vi "FlexRIO_CPUIMAQ.vi"() -> ()   [LabVIEW 2013]
uses:
  <vilib>/rvi/Emulation/niFpgaSctlEmulationGetInTimedLoop.vi
  <vilib>/rvi/Emulation/niFpgaEmulationReportErrorSimple.vi
  <vilib>/rvi/Emulation/niFpgaGetClockAttributes.vi
  <vilib>/rvi/interface/RandomDataEmulation/nirviRandomDataFPGAFIFO.vi
  <vilib>/rvi/interface/RandomDataEmulation/niFpgaRandomDataHandleErrors.vi
  <vilib>/rvi/Emulation/niFpgaCriticalErrorInLSC.vi
  <vilib>/rvi/DataTransferAndStorage/Container/XNode/niFpgaContainer.xnode
  <vilib>/rvi/interface/RandomDataEmulation/nirviRandomDataFpgaReadWriteTemplate.vi
panel:
  out "uartOverrunError":bool
  out "uartFramingError":bool
  out "uartBreakIndicator":bool
  out "uartRxByte":u8 format="%02x"
  out "uartTxReady":bool
  out "uartRxReady":bool
  in  "uartTxByte":u8=1 format="%x"
  in  "uartByteMode":bool=TRUE
  in  "uartBaudRate":u8=1
  in  "uartSetBaudRate":bool
  in  "uartReceive":bool
  in  "uartTransmit":bool
  in  "ControlEnable":bool=TRUE
  in  "LineScan":bool
  in  "SpareHigh":bool=TRUE
  in  "LVALHigh":bool=TRUE
  in  "FVALHigh":bool=TRUE
  in  "DVALHigh":bool=TRUE
  in  "SignalMapping":u8(ring) items=["Standard", "Basler 10 tap", "Vosskühler 10 tap"]
  in  "Configuration":u8(ring)=2 items=["Base", "Medium", "Full/Extended"]
  out "PXIIN1":bool
  in  "PXIOUT1":bool
  out "PXIIN0":bool
  in  "PXIOUT0":bool
  out "auxDI1":bool
  out "auxDI0":bool
  out "DI1":bool
  out "DI0":bool
  in  "auxDO1":bool
  in  "auxDO0":bool
  in  "DO1":bool
  in  "DO0":bool
  in  "auxAO1":i32
  in  "auxAO0":i32
  out "auxAI1":i32
  out "auxAI0":i32
  out "DMATtoHOSTOverflows":u16
  in  "DMATtoHOSTEnable0":bool
  out "DMATtoHOSTSampleSize":u8[](array[numeric])
  out "DMATtoHOSTFrameType":u8[](array[numeric])
  out "DMATtoHOSTNCh":u16[](array[numeric])
  out "Platform":enum8{"FlexRIO", "cRIO", "RSeries"}(ring)
  in  "DebugMode":bool
  in  "DAQStartStop":bool
  out "DevProfile":T1(ring)=enum."CPUImage"
  out "DevTemp":i16=-10244
  out "DevQualityStatus":u8
  out "Fref":u32=100000000
  out "RIOAdapterCorrect":bool=TRUE
  out "InsertedIOModule ID":u32
  out "InitDone":bool=TRUE
  out "FPGAVIversion":u8[](array[numeric])=[1, 0]
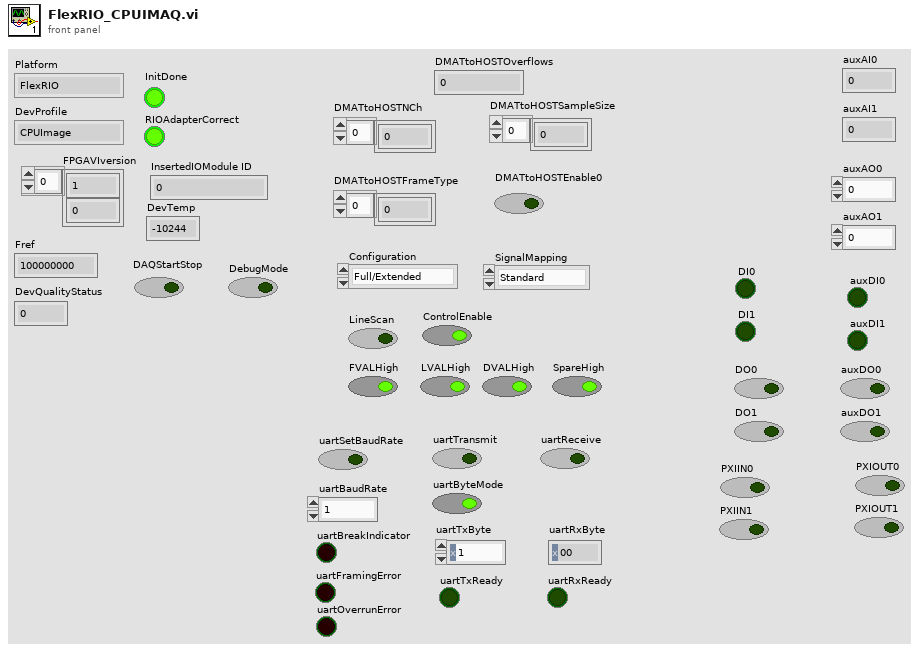
[diagram p1: front panel]
types:
  T1 = enum8{"CPUData", "CPUImage", "GPUData", "GPUImage"}
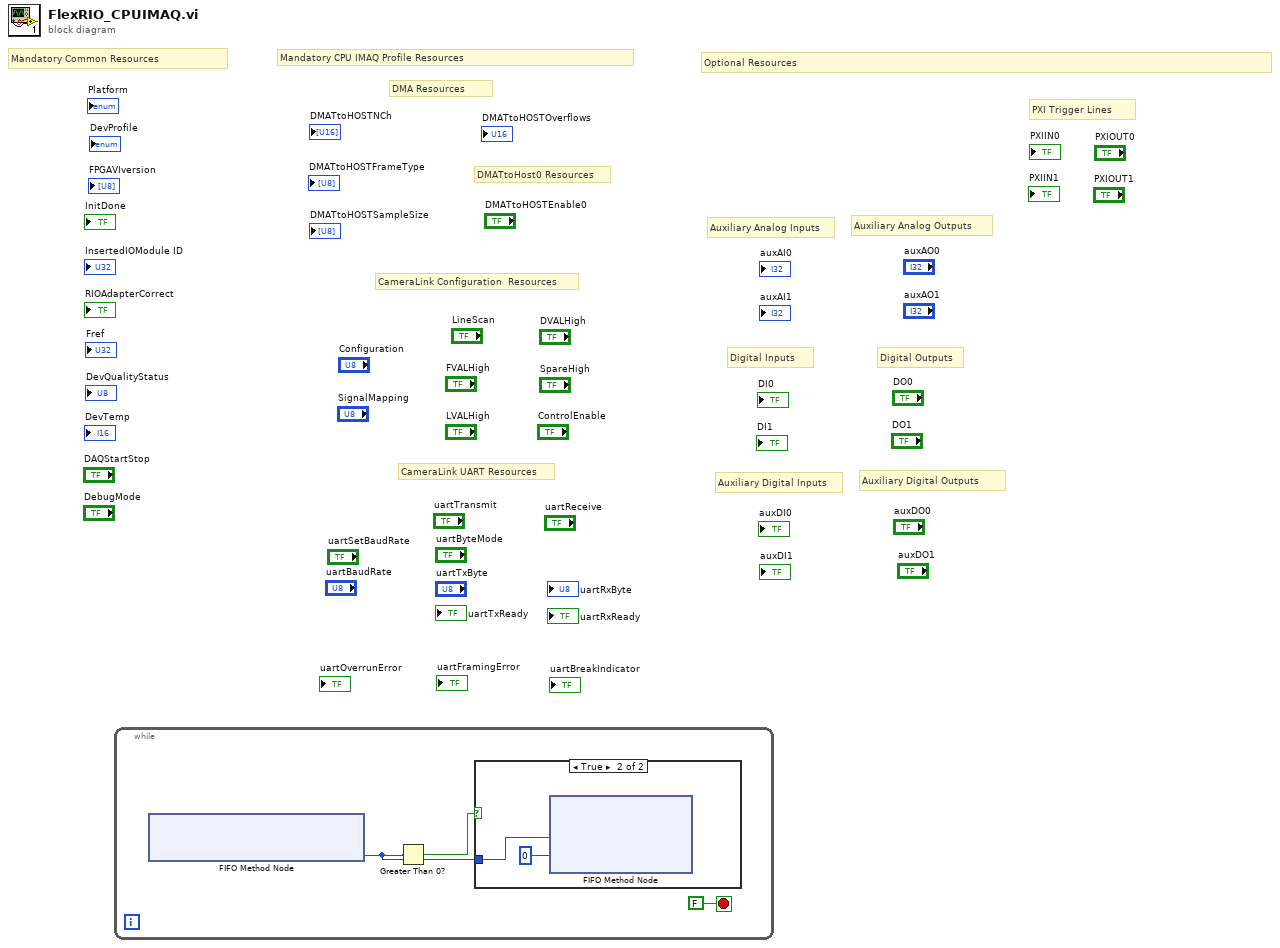
[diagram p0: block diagram]
diagram:
  # "CameraLink UART Resources"
  # "CameraLink Configuration  Resources"
  # "DMA Resources"
  # "PXI Trigger Lines"
  # "Digital Outputs"
  # "Auxiliary Digital Outputs"
  # "Auxiliary Digital Inputs"
  # "Digital Inputs"
  # "Auxiliary Analog Outputs"
  # "Auxiliary Analog Inputs"
  # "Optional Resources"
  # "DMATtoHost0 Resources"
  # "Mandatory CPU IMAQ Profile Resources"
  # "Mandatory Common Resources"
  n1 = while {
    stop <- FALSE stop-if-true
    n2 = xnode ("FIFO Method Node")() -> ("Number of Elements to Write"=w1:u32)  [unwired: 1 in, 1 out]
    n3 = Greater Than 0?(x=w1) -> (x > 0?=w2:bool)
    n4 = case shown="True" w2 {
      tunnel: w1 -> [_ w5]
      frame False {
      }
      frame True {
        n5 = xnode ("FIFO Method Node")("Element"=w5, "Timeout"=i16 0) -> ()  [unwired: 1 in, 2 out]
      }
    }
  }
